vi "try_Conditional Highlight Execution.vi"() -> ()   [LabVIEW 2020]
uses:
  <vilib>/gmath/NI_Gmath.lvlib
  <vilib>/gmath/statdist.llb/Normal Random.vi
  <vilib>/gmath/statdist.llb/Uniform Random.vi
  <vilib>/Analysis/NI_AALPro.lvlib
panel:
  in  "Variable 1":u16(ring)=2 items=["None", "Gaussian", "Uniform"]
  in  "Variable 3":u16(ring) items=["None", "Gaussian", "Uniform"]
  in  "Variable 2":u16(ring) items=["None", "Gaussian", "Uniform"]
  out "Waveform Graph":dbl[](graph)
  in  "Probability Samples":i32=50
  in  "Samples/iteration":i32=5000
  out "Cumulative Density Function (CDF)":cluster{"Ramp Pattern":dbl[], dbl[]}(graph)
  out "Probability Density Function (PDF)":cluster{"Ramp Pattern":dbl[], dbl[]}(graph)
  # "Conditional Highlight Execution Demo"
  # "See the block diagram."
  # "Close this VI when you are done with the demo."
  # "You do not need to save changes to this VI."
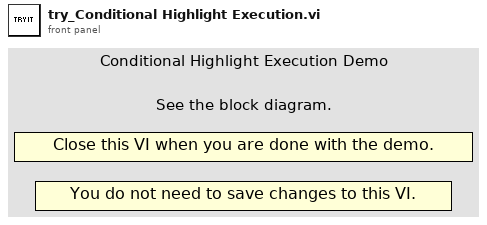
[diagram p1: front panel]
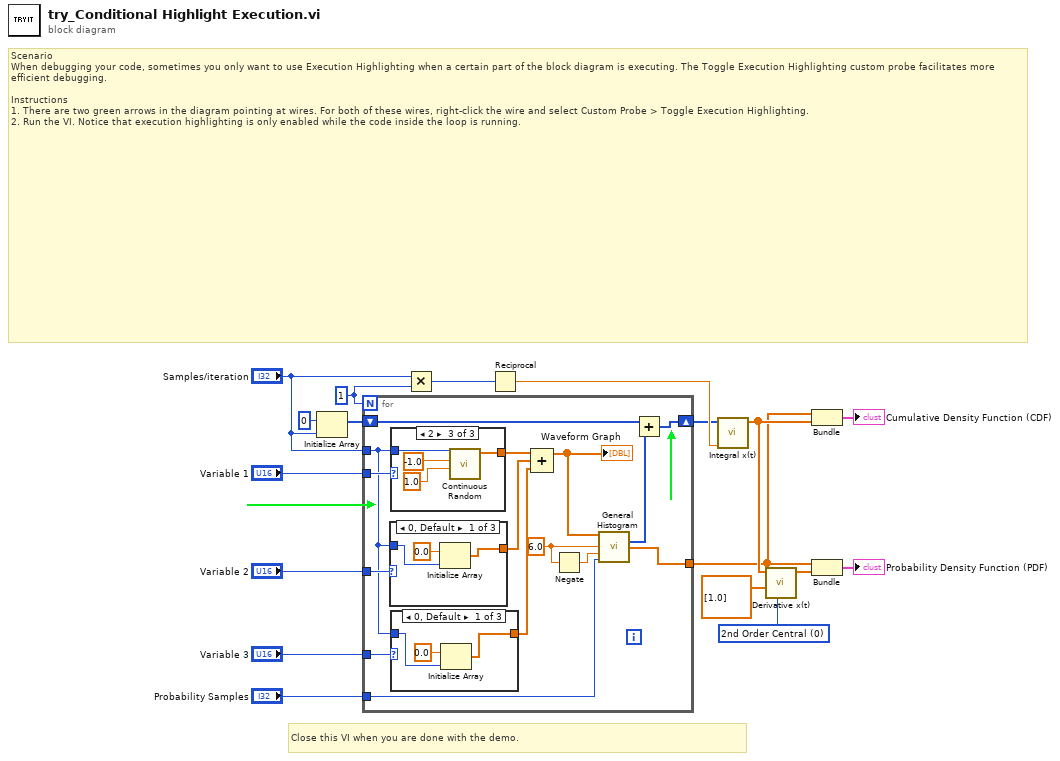
[diagram p0: block diagram]
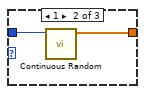
[diagram p2: hidden frame]
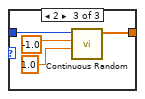
[diagram p3: hidden frame]
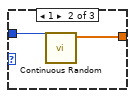
[diagram p4: hidden frame]
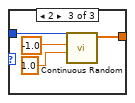
[diagram p5: hidden frame]
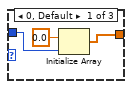
[diagram p6: hidden frame]
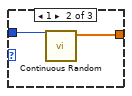
[diagram p7: hidden frame]
diagram:
  w3 = 1 ("# of iterations")
  w9 = u16 0 items=["2nd Order Central", "4th Order Central", "Forward", "Backward"] ("method")
  # "Close this VI when you are done with the demo."
  # "Scenario\nWhen debugging your code, sometimes you only want to use Execution Highlighting when a certain part of the block diagram is executing. The Toggle Execution Highlighting custom probe facilitates more efficient debugging.\n\nInstructions\n1. There are two green arrows in the diagram pointing at wires. For both of these wires, right-click the wire and select Custom Probe > Toggle Execution Highlighting.\n2. Run the VI. Notice that execution highlighting is only enabled while the code inside the loop is running."
  n1 = Initialize Array(0 ("initialized array"), "Samples/iteration") -> (w18:i32[])
  n2 = for {
    N: w3 -> [_]
    shift-right: [w31] -> w8
    shift-left: w18 -> [w32]
    tunnel: "Samples/iteration" -> [w24]
    tunnel: "Probability Samples" -> [w33]
    tunnel: [w30] -> w7
    tunnel: "Variable 2" -> [w26]
    tunnel: "Variable 1" -> [w27]
    tunnel: "Variable 3" -> [w25]
    w23 = 6.0 ("max")
    # "Iterate the histogram several times to make the PDF and CDF approximate the ideal distribution."
    n3 = case shown="0, Default" w26 {
      tunnel: w24 -> [w44 w47 w51]
      tunnel: [w45 w46 w50] -> w20
      frame 0, Default {
        n4 = Initialize Array(0.0 ("element"), w44) -> (w45:dbl[])
      }
      frame 1 {
        n5 = call-poly <vilib>:"Continuous Random.vi"("samples"=w47) -> ("normal random data"=w46:dbl[])  [unwired: 9 in, 1 out]
      }
      frame 2 {
        n6 = call-poly <vilib>:"Continuous Random.vi"("xmax"=1.0, "xmin"=-1.0, "samples"=w51) -> ("uniform random data"=w50:dbl[])  [unwired: 7 in, 1 out]
      }
    }
    n7 = case shown="2" w27 {
      tunnel: w24 -> [w53 w56 w60]
      tunnel: [w54 w55 w59] -> w19
      frame 0, Default {
        n8 = Initialize Array(0.0 ("element"), w53) -> (w54:dbl[])
      }
      frame 1 {
        n9 = call-poly <vilib>:"Continuous Random.vi"("samples"=w56) -> ("normal random data"=w55:dbl[])  [unwired: 9 in, 1 out]
      }
      frame 2 {
        n10 = call-poly <vilib>:"Continuous Random.vi"("xmax"=1.0, "xmin"=-1.0, "samples"=w60) -> ("uniform random data"=w59:dbl[])  [unwired: 7 in, 1 out]
      }
    }
    n11 = case shown="0, Default" w25 {
      tunnel: w24 -> [w35 w38 w42]
      tunnel: [w36 w37 w41] -> w21
      frame 0, Default {
        n12 = Initialize Array(0.0 ("element"), w35) -> (w36:dbl[])
      }
      frame 1 {
        n13 = call-poly <vilib>:"Continuous Random.vi"("samples"=w38) -> ("normal random data"=w37:dbl[])  [unwired: 9 in, 1 out]
      }
      frame 2 {
        n14 = call-poly <vilib>:"Continuous Random.vi"("xmax"=1.0, "xmin"=-1.0, "samples"=w42) -> ("uniform random data"=w41:dbl[])  [unwired: 7 in, 1 out]
      }
    }
    n15 = Compound Arithmetic op=ADD(w19, w20, w21) -> (w28:dbl[])
    "Waveform Graph" <- w28
    n16 = Negate(x=w23) -> (-x=w22:dbl)
    n17 = call <vilib>:"General Histogram.vi"("X"=w28, "max"=w23, "min"=w22, "# bins"=w33) -> ("Histogram"=w29:i32[], "Axis"=w30:dbl[])  [unwired: 7 in, 3 out]
    n18 = Add(x=w32, y=w29) -> (x+y=w31:i32[])
  }
  n19 = Multiply(x="Samples/iteration", y=w3) -> (x*y=w2:i32)
  n20 = Reciprocal(x=w2) -> (1/x=w12:dbl)
  n21 = call <vilib>:"Integral x(t).vi"("dt"=w12, "X"=w8) -> ("Integral X"=w16:dbl[])  [unwired: 8 in, 1 out]
  n22 = call <vilib>:"Derivative x(t).vi"("method"=w9, "Final Condition"=dbl[] [1.0] ("final condition"), "X"=w16) -> ("dX/dt"=w15:dbl[])  [unwired: 7 in, 1 out]
  n23 = Bundle("Axis"=w7, "Integral X"=w16) -> (→"Cumulative Density Function (CDF)":cluster{"Axis":dbl[], "Integral X":dbl[]})  [unwired: 1 in]
  n24 = Bundle("Axis"=w7, "dX/dt"=w15) -> (→"Probability Density Function (PDF)":cluster{"Axis":dbl[], "dX/dt":dbl[]})  [unwired: 1 in]
